vi "write aviatif file (SubVI).vi"(8 "error in":errorcluster, 10 "img data":u16[][][][](array[numeric]), 11 "path":path) -> (0 "error out":errorcluster)   [LabVIEW 2024]
panel:
  out "concatenated string":string
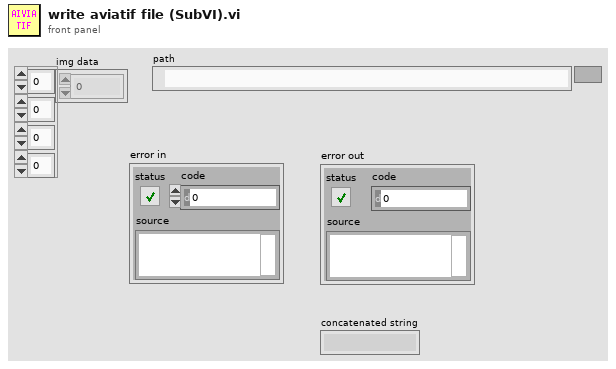
[diagram p1: front panel]
types:
  T1 = cluster{"Unit":enum16{"undefined", "host depend", "inch", "cm"}, "X":cluster{"Pixels":u32, "Units":u32}, "Y":cluster{"Pixels":u32, "Units":u32}}
  T2 = typedef "imagedata.ctl" = cluster{"image type":i32, "image depth":i32, "image":u8[], "mask":u8[], "colors":u32[], "Rectangle":cluster{"left":i16, "top":i16, "right":i16, "bottom":i16}}
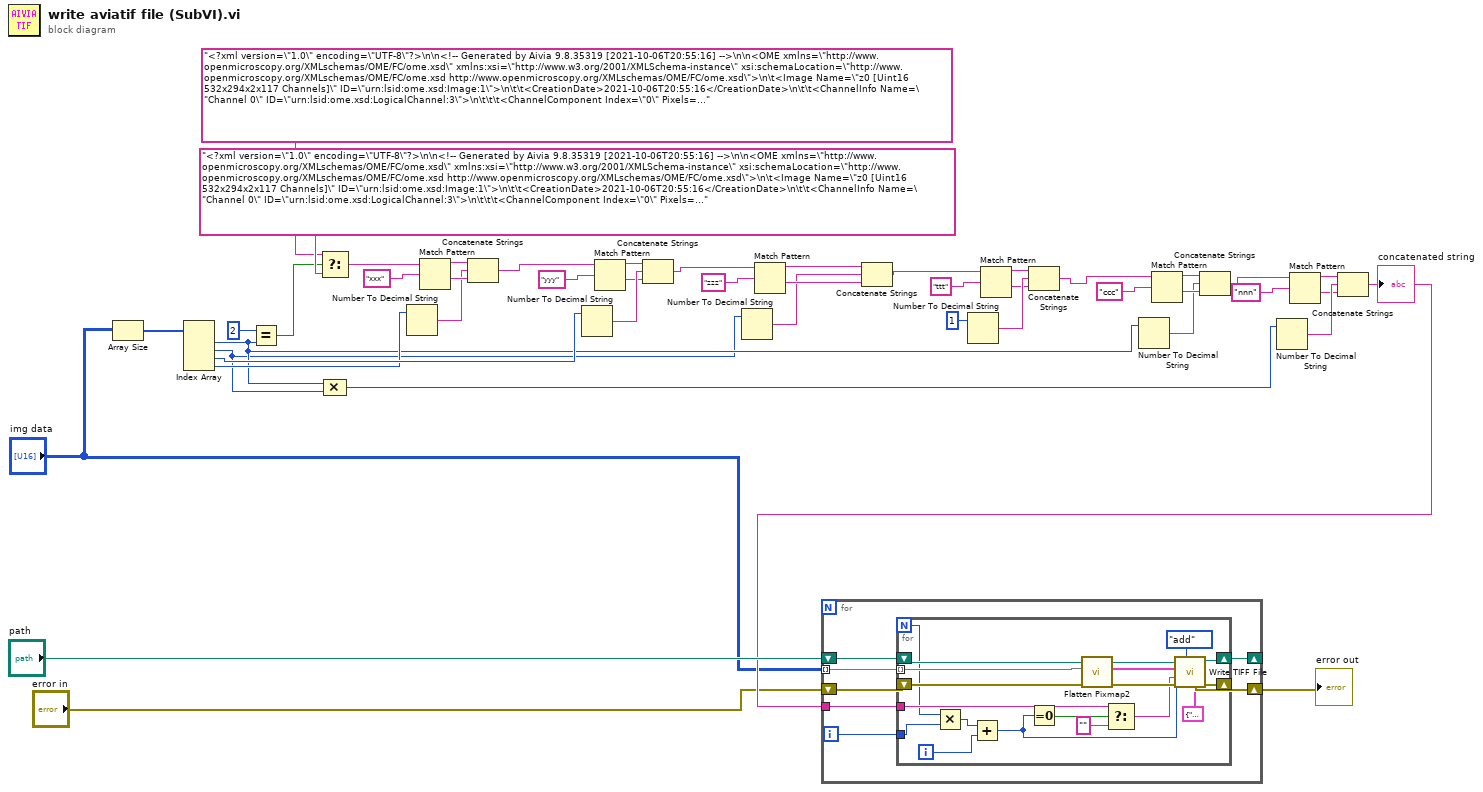
[diagram p0: block diagram]
diagram:
  n1 = Array Size(array="img data") -> (size(s)=w9:i32[])
  n2 = Index Array(array=w9) -> (element #1=w3:i32, element #2=w2:i32, element #3=w11:i32, element #4=w10:i32)  [unwired: 4 in]
  n3 = Equal?(x=2, y=w3) -> (x = y?=w13:bool)
  n4 = Select(t="<?xml version=\"1.0\" encoding=\"UTF-8\"?>\n\n<!-- Generated by Aivia 9.8.35319 [2021-10-06T20:55:16] -->\n\n<OME xmlns=\"http://www.openmicroscopy.org/XMLschemas/OME/FC/ome.xsd\" xmlns:xsi=\"http://www.w3.org/2001/XMLSchema-instance\" xsi:schemaLocation=\"http://www.openmicroscopy.org/XMLschemas/OME/FC/ome.xsd http://www.openmicroscopy.org/XMLschemas/OME/FC/ome.xsd\">\n\t<Image Name=\"z0 [Uint16 532x294x2x117 Channels]\" ID=\"urn:lsid:ome.xsd:Image:1\">\n\t\t<CreationDate>2021-10-06T20:55:16</CreationDate>\n\t\t<ChannelInfo Name=\"Channel 0\" ID=\"urn:lsid:ome.xsd:LogicalChannel:3\">\n\t\t\t<ChannelComponent Index=\"0\" Pixels=\"urn:lsid:ome.xsd:Pixels:2\"/>\n\t\t</ChannelInfo>\n\t\t<ChannelInfo Name=\"Channel 1\" ID=\"urn:lsid:ome.xsd:LogicalChannel:4\">\n\t\t\t<ChannelComponent Index=\"1\" Pixels=\"urn:lsid:ome.xsd:Pixels:2\"/>\n\t\t</ChannelInfo>\n\t\t<Pixels DimensionOrder=\"XYZTC\" PixelType=\"Uint16\" SizeX=\"xxx\" SizeY=\"yyy\" SizeZ=\"zzz\" SizeT=\"ttt\" SizeC=\"ccc\" BigEndian=\"false\" ID=\"urn:lsid:ome.xsd:Pixels:2\">\n\t\t\t<TiffData IFD=\"0\" NumPlanes=\"nnn\"/>\n\t\t</Pixels>\n\t</Image>\n</OME>", s=w13, f="<?xml version=\"1.0\" encoding=\"UTF-8\"?>\n\n<!-- Generated by Aivia 9.8.35319 [2021-10-06T20:55:16] -->\n\n<OME xmlns=\"http://www.openmicroscopy.org/XMLschemas/OME/FC/ome.xsd\" xmlns:xsi=\"http://www.w3.org/2001/XMLSchema-instance\" xsi:schemaLocation=\"http://www.openmicroscopy.org/XMLschemas/OME/FC/ome.xsd http://www.openmicroscopy.org/XMLschemas/OME/FC/ome.xsd\">\n\t<Image Name=\"z0 [Uint16 532x294x2x117 Channels]\" ID=\"urn:lsid:ome.xsd:Image:1\">\n\t\t<CreationDate>2021-10-06T20:55:16</CreationDate>\n\t\t<ChannelInfo Name=\"Channel 0\" ID=\"urn:lsid:ome.xsd:LogicalChannel:3\">\n\t\t\t<ChannelComponent Index=\"0\" Pixels=\"urn:lsid:ome.xsd:Pixels:2\"/>\n\t\t</ChannelInfo>\n\t\t<ChannelInfo Name=\"Channel 1\" ID=\"urn:lsid:ome.xsd:LogicalChannel:4\">\n\t\t\t<ChannelComponent Index=\"1\" Pixels=\"urn:lsid:ome.xsd:Pixels:2\"/>\n\t\t</ChannelInfo>\n\t\t<Pixels DimensionOrder=\"XYZTC\" PixelType=\"Uint16\" SizeX=\"xxx\" SizeY=\"yyy\" SizeZ=\"zzz\" SizeT=\"ttt\" SizeC=\"ccc\" BigEndian=\"false\" ID=\"urn:lsid:ome.xsd:Pixels:2\">\n\t\t\t<TiffData IFD=\"0\" NumPlanes=\"nnn\"/>\n\t\t</Pixels>\n\t</Image>\n</OME>") -> (s? t:f=w41:string)
  n5 = Compound Arithmetic op=MULTIPLY(w3, w2) -> (w1:i32)
  n6 = Number To Decimal String(number=w10) -> (decimal integer string=w40:string)  [unwired: 1 in]
  n7 = Match Pattern(string=w41, regular expression="xxx") -> (before substring=w44:string, after substring=w45:string)  [unwired: 1 in, 2 out]
  n8 = Concatenate Strings(w44, w40, w45) -> (w19:string)
  n9 = Number To Decimal String(number=w11) -> (decimal integer string=w39:string)  [unwired: 1 in]
  n10 = Match Pattern(string=w19, regular expression="yyy") -> (before substring=w38:string, after substring=w37:string)  [unwired: 1 in, 2 out]
  n11 = Concatenate Strings(w38, w39, w37) -> (w18:string)
  n12 = Number To Decimal String(number=w2) -> (decimal integer string=w32:string)  [unwired: 1 in]
  n13 = Match Pattern(string=w18, regular expression="zzz") -> (before substring=w33:string, after substring=w34:string)  [unwired: 1 in, 2 out]
  n14 = Concatenate Strings(w33, w32, w34) -> (w17:string)
  n15 = Number To Decimal String(number=1) -> (decimal integer string=w31:string)  [unwired: 1 in]
  n16 = Match Pattern(string=w17, regular expression="ttt") -> (before substring=w30:string, after substring=w29:string)  [unwired: 1 in, 2 out]
  n17 = Concatenate Strings(w30, w31, w29) -> (w16:string)
  n18 = Number To Decimal String(number=w3) -> (decimal integer string=w24:string)  [unwired: 1 in]
  n19 = Match Pattern(string=w16, regular expression="ccc") -> (before substring=w25:string, after substring=w26:string)  [unwired: 1 in, 2 out]
  n20 = Concatenate Strings(w25, w24, w26) -> (w15:string)
  n21 = Number To Decimal String(number=w1) -> (decimal integer string=w23:string)  [unwired: 1 in]
  n22 = Match Pattern(string=w15, regular expression="nnn") -> (before substring=w22:string, after substring=w21:string)  [unwired: 1 in, 2 out]
  n23 = Concatenate Strings(w22, w23, w21) -> (w7:string)
  "concatenated string" <- w7
  n24 = for {
    tunnel: w7 -> [w52]
    shift-right: [w51] -> _
    shift-left: "path" -> [w53]
    tunnel: "img data" -> [w50] mode=indexing
    shift-right: [w48] -> w4
    shift-left: "error in" -> [w49]
    i -> [w47]
    n25 = for {
      N -> [w57]
      shift-right: [w68] -> w51
      shift-left: w53 -> [w69]
      shift-right: [w66] -> w48
      shift-left: w49 -> [w67]
      tunnel: w52 -> [w64]
      tunnel: w50 -> [w59] mode=indexing
      tunnel: w47 -> [w58]
      i -> [w55]
      n26 = Multiply(x=w57, y=w58) -> (x*y=w56:i32)
      n27 = Add(x=w56, y=w55) -> (x+y=w54:i32)
      n28 = Equal To 0?(x=w54) -> (x = 0?=w65:bool)
      n29 = call "Flatten Pixmap2.vi"("16-bit pixmap"=w59) -> ("image data"=w60:T2)  [unwired: 10 in]
      n30 = Select(t=w64, s=w65, f="") -> (s? t:f=w62:string)
      n31 = call "Write TIFF File.vi"("Resolution"=T1 {"Unit"=enum."host depend", "X"={"Pixels"=0, "Units"=1}, "Y"={"Pixels"=0, "Units"=1}}, "Position"=w54, "mode"=enum16{"replace", "add"}."add", "エラー入力（エラーなし）"=w67, "ImageDescription"=w62, "image data"=w60, "path to TIFF file"=w69) -> ("エラー出力"=w66:errorcluster, "path"=w68:path)  [unwired: 3 in]
    }
  }
  "error out" <- w4
